vi "Generate Texture Array And Data.vi"(8 "y":i32, 9 "x":i32, 10 "Texture":T2, 11 "output cluster":T3) -> (0 "P3 Mapped":T1, 1 "P2 Mapped":T1, 2 "P1 Mapped":T1, 3 "Array":u32[][](array[numeric]), 4 "x step":i32, 6 "y step":i32)   [LabVIEW 2022 SP3, in "Raster.lvlib"]
uses:
  Raster.lvlib
  Point 2D.ctl
  <vilib>/picture/picture.llb/imagedata.ctl
  Utility/Convert Pixels To Picture.vi/d601d993-a776-4dc8-89c7-357d8398c88c.vi
  Utility/Convert Pixels To Picture.vi/7816d0d6-8e4d-41a2-85ac-ed82f1435763.vi
  <vilib>/Utility/High Resolution Relative Seconds.vi
  <vilib>/picture/picture.llb/Draw Unflattened Pixmap.vi
  <vilib>/picture/picture.llb/Draw True-Color Pixmap.vi
  Utility/Utility.lvlib
panel:
  out "2D Picture 2":picture
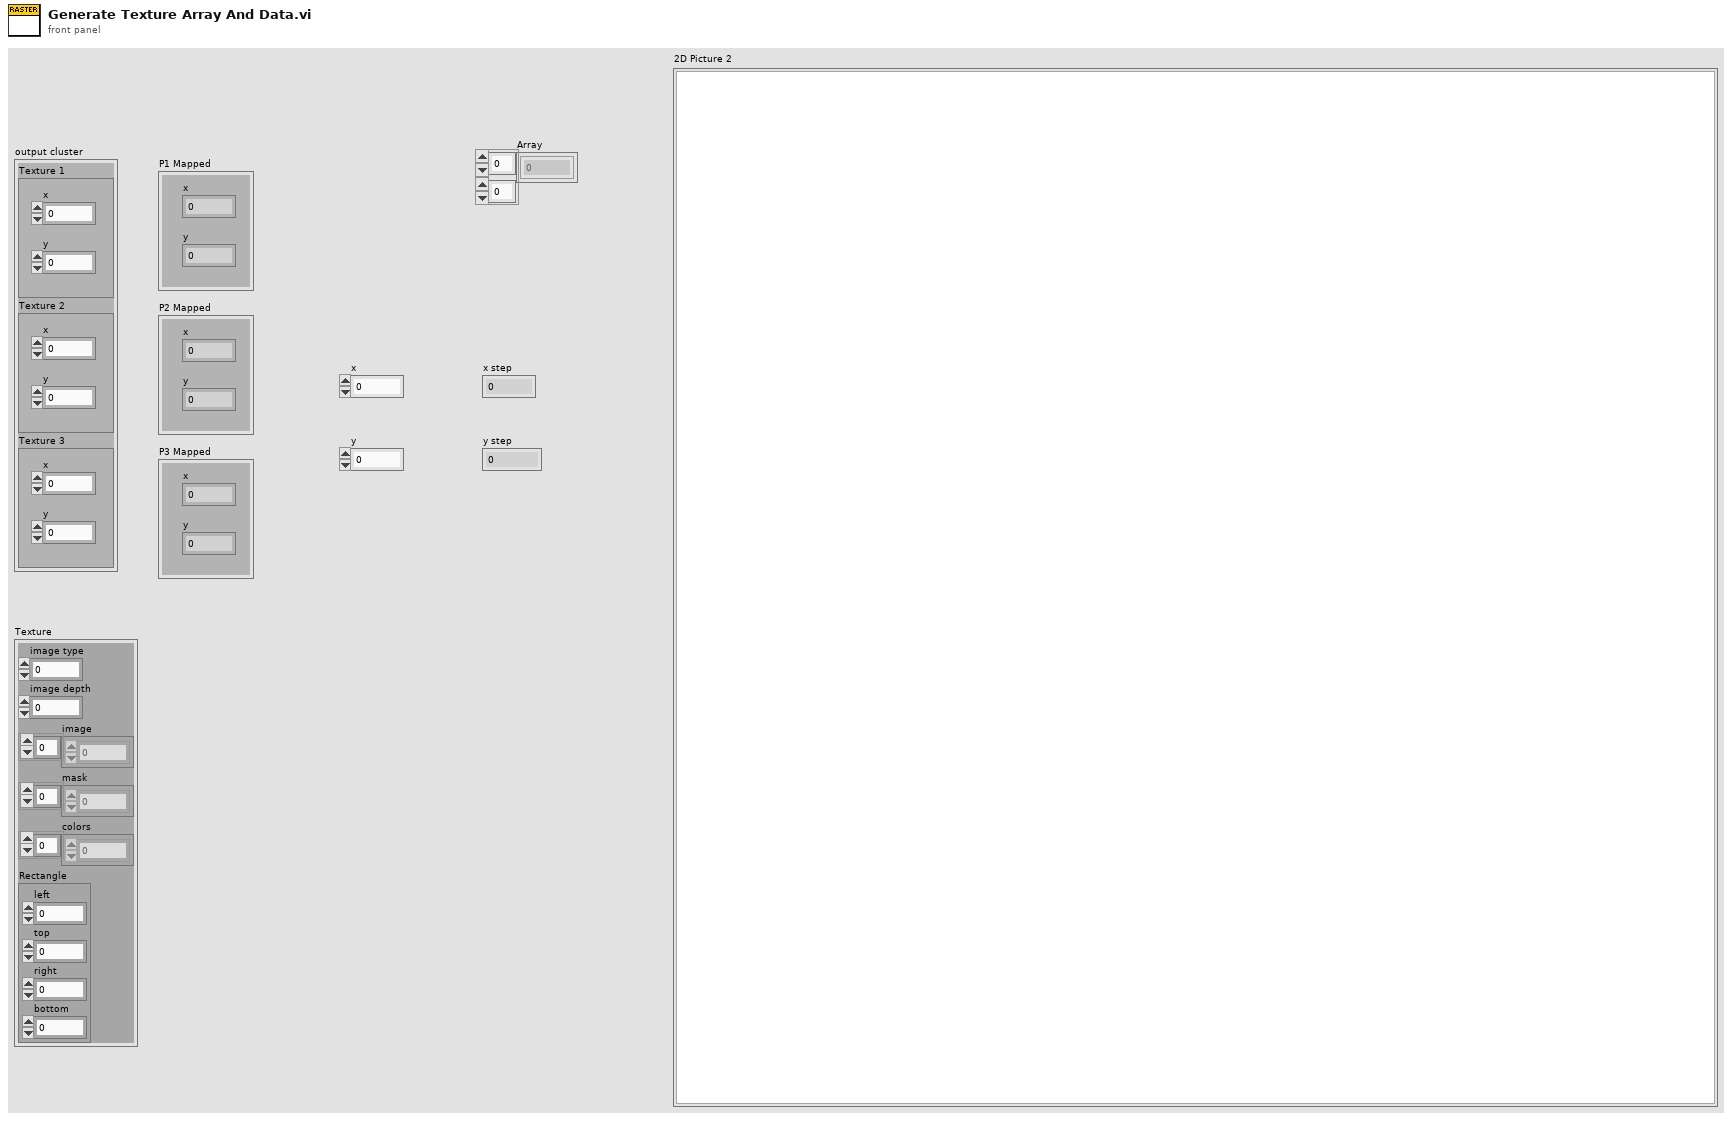
[diagram p1: front panel]
types:
  T1 = typedef "Raster.lvlib/Point 2D.ctl" = cluster{"x":i32, "y":i32}
  T2 = typedef "imagedata.ctl" = cluster{"image type":i32, "image depth":i32, "image":u8[], "mask":u8[], "colors":u32[], "Rectangle":cluster{"left":i16, "top":i16, "right":i16, "bottom":i16}}
  T3 = cluster{"Texture 1":T1, "Texture 2":T1, "Texture 3":T1}
  T4 = cluster{"left":i16, "top":i16, "right":i16, "bottom":i16}
  T5 = cluster{"left":i32, "top":i32, "right":i32, "bottom":i32}
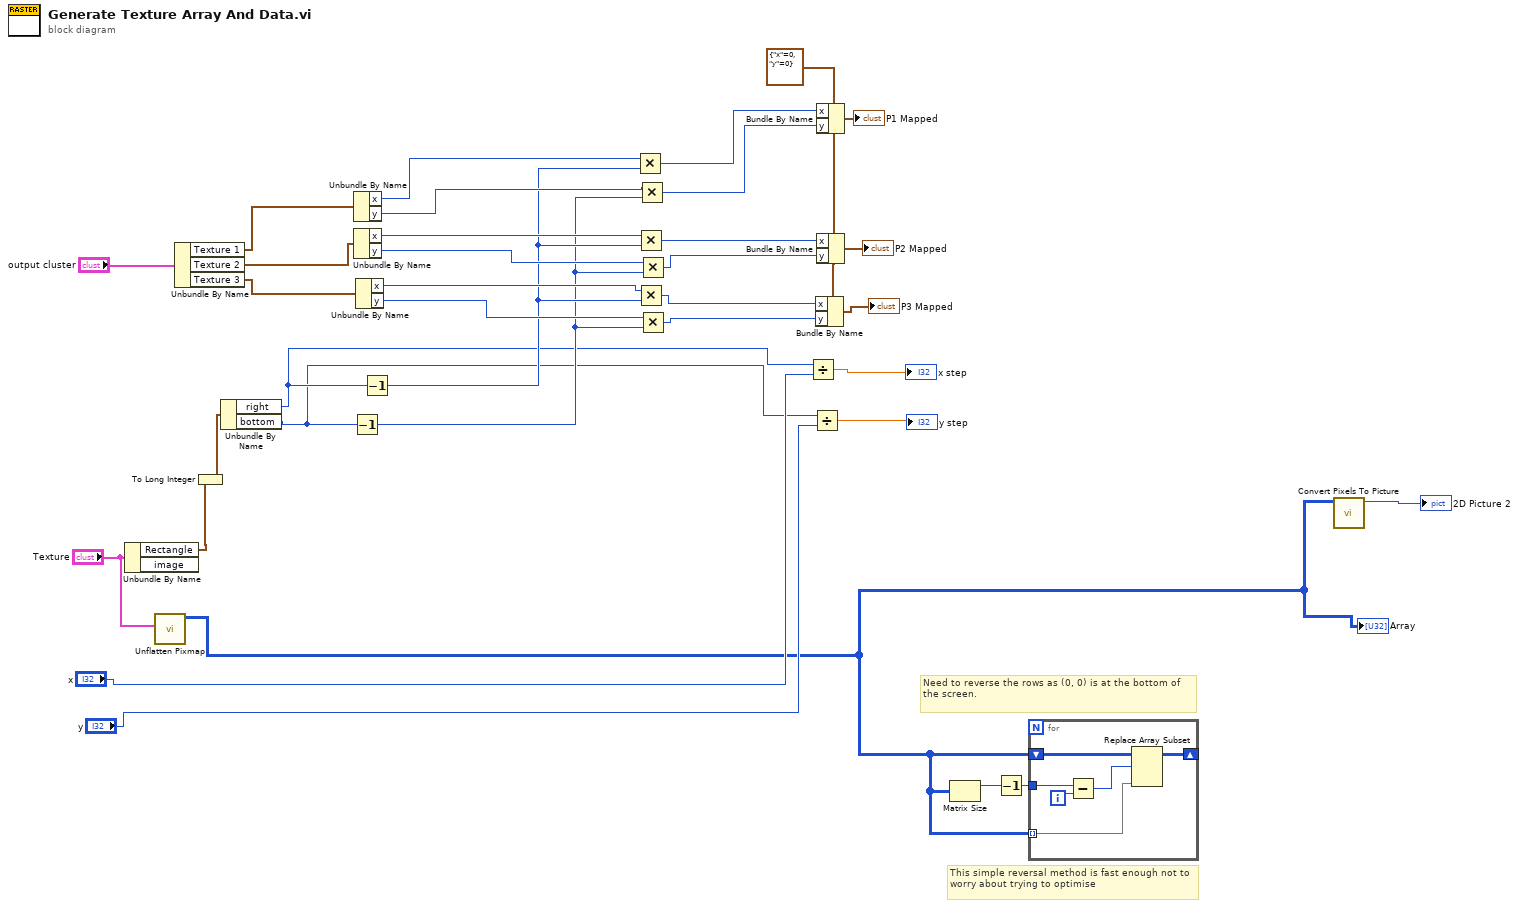
[diagram p0: block diagram]
diagram:
  w15 = T1 {"x"=0, "y"=0} ("Texture 1")
  # "Need to reverse the rows as (0, 0) is at the bottom of the screen."
  # "This simple reversal method is fast enough not to worry about trying to optimise"
  n1 = Unbundle By Name("Texture") -> ("Rectangle"=w31:T4)  [unwired: 1 out]
  n2 = call <vilib>:"Unflatten Pixmap.vi"("image data"="Texture") -> ("24-bit pixmap"=w1:u32[][])  [unwired: 4 in, 6 out]
  "Array" <- w1
  n3 = Unbundle By Name("output cluster") -> ("Texture 1"=w33:T1, "Texture 2"=w34:T1, "Texture 3"=w35:T1)
  n4 = To Long Integer(number=w31) -> (32bit integer=w28:T5)
  n5 = Unbundle By Name(w28) -> ("right"=w9:i32, "bottom"=w8:i32)
  n6 = Decrement(x=w8) -> (x-1=w12:i32)
  n7 = Unbundle By Name(w33) -> ("x"=w30:i32, "y"=w29:i32)
  n8 = Unbundle By Name(w34) -> ("x"=w27:i32, "y"=w26:i32)
  n9 = Unbundle By Name(w35) -> ("x"=w25:i32, "y"=w24:i32)
  n10 = Decrement(x=w9) -> (x-1=w13:i32)
  n11 = Multiply(x=w30, y=w13) -> (x*y=w23:i32)
  n12 = Multiply(x=w27, y=w13) -> (x*y=w20:i32)
  n13 = Multiply(x=w25, y=w13) -> (x*y=w17:i32)
  n14 = Multiply(x=w29, y=w12) -> (x*y=w22:i32)
  n15 = Multiply(x=w26, y=w12) -> (x*y=w19:i32)
  n16 = Multiply(x=w24, y=w12) -> (x*y=w16:i32)
  n17 = Divide(x=w9, y="x") -> (x/y=→"x step":dbl)
  n18 = Divide(x=w8, y="y") -> (x/y=→"y step":dbl)
  n19 = Bundle By Name(cluster=w15, "x"=w17, "y"=w16) -> (→"P3 Mapped":T1)
  n20 = Bundle By Name(cluster=w15, "x"=w23, "y"=w22) -> (→"P1 Mapped":T1)
  n21 = Bundle By Name(cluster=w15, "x"=w20, "y"=w19) -> (→"P2 Mapped":T1)
  n22 = Matrix Size(0:w1) -> (1:w3:i32)  [unwired: 1 out]
  n23 = Decrement(x=w3) -> (x-1=w4:i32)
  n24 = for {
    tunnel: w1 -> [w37] mode=indexing
    shift-right: [w36] -> _
    shift-left: w1 -> [w41]
    tunnel: w4 -> [w40]
    i -> [w39]
    n25 = Subtract(x=w40, y=w39) -> (x-y=w38:i32)
    n26 = Replace Array Subset(array=w41, new element=w37, index (row)=w38) -> (w36:u32[][])  [unwired: 1 in]
  }
  n27 = call "Convert Pixels To Picture.vi"("Pixel Data in"=w1) -> ("2D Picture"=→"2D Picture 2":picture)  [unwired: 9 in, 1 out]
